vi "AVS_SuppressStrayLight.vi"(4 "a_pDestSpectrum":dbl[](array[numeric]), 5 "a_pSrcSpectrum":dbl[](array[numeric]), 6 "a_Multifactor":sgl, 7 "a_hDevice":i32) -> (0 "a_pDestSpectrum":dbl[](array[numeric]), 1 "a_pSrcSpectrum":dbl[](array[numeric]), 3 "Output Value":i32)   [LabVIEW 2016]
uses:
  libavs.so
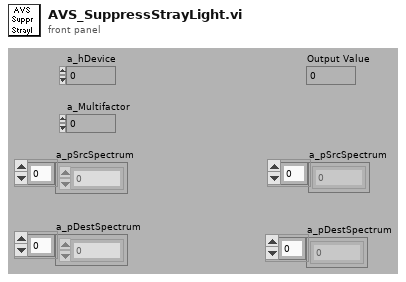
[diagram p1: front panel]
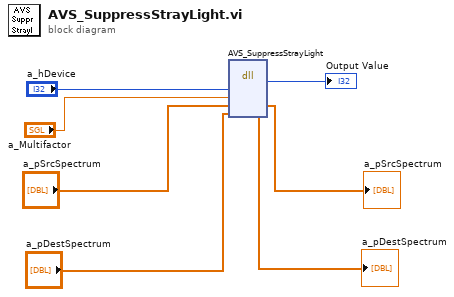
[diagram p0: block diagram]
diagram:
  n1 = dll-call lib="home/harini/tcs/ts_sedspectrometer/ss_sedspectrometer/VIs/libavs.so" fn="AVS_SuppressStrayLight"("a_hDevice"="a_hDevice", "a_Multifactor"="a_Multifactor", "a_pSrcSpectrum"="a_pSrcSpectrum", "a_pDestSpectrum"="a_pDestSpectrum") -> ("return type"=→"Output Value":i32, "a_pSrcSpectrum"=→"a_pSrcSpectrum":dbl[], "a_pDestSpectrum"=→"a_pDestSpectrum":dbl[])  [unwired: 5 in, 2 out]
